vi "Initialize with Topology.vi"   [LabVIEW 2020, in "SLSC Switch.lvlib"]
doc: "Returns a session handle used to identify the SLSC Switch module in all subsequent driver calls and sets the topology of the switch module."
uses:
  <vilib>/SLSC_Switch/SLSC Switch.lvlib
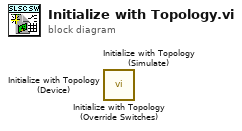
[diagram p0: block diagram]
diagram:
  n1 = call <vilib>:"Initialize with Topology (Override Switches).vi"() -> ()  [unwired: 10 in, 2 out]
  n2 = call <vilib>:"Initialize with Topology (Simulate).vi"() -> ()  [unwired: 10 in, 2 out]
  n3 = call <vilib>:"Initialize with Topology (Device).vi"() -> ()  [unwired: 10 in, 2 out]
